vi "Create Logger.vi"(8 "error in (no error)":errorcluster, 11 "Logger.Error in":refnum<class "Logger.Error.lvclass">) -> (0 "error out":errorcluster, 3 "Logger.Error out":refnum<class "Logger.Error.lvclass">)   [LabVIEW 2016, in "Logger.Error.lvclass"]
uses:
  Logger.Error.lvclass
  <userlib>/_MGI/Error Reporter/MGI Error Reporter Base/MGI Error Reporter Base.lvclass
  <userlib>/_MGI/Error Reporter/MGI Error Reporter Dialog/MGI Error Reporter Dialog.lvclass
  Logger/Logger.lvclass
  C:/Program Files (x86)/National Instruments/LabVIEW 2016/user.lib/_MGI/Error Reporter/MGI Error Reporter Base/MGI Error Reporter Base.lvclass
panel:
  out "Already Running?":bool
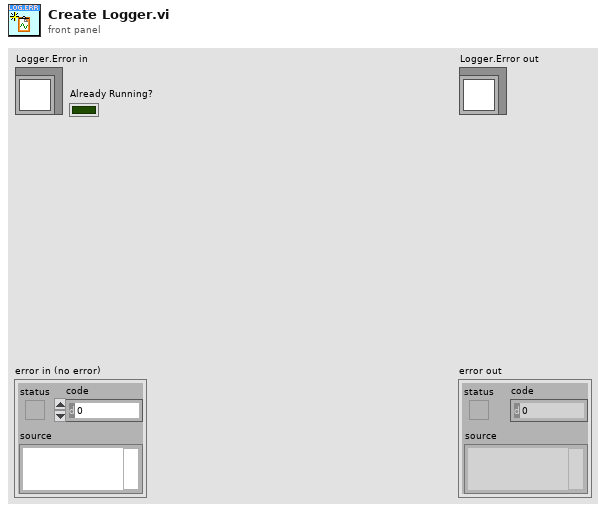
[diagram p1: front panel]
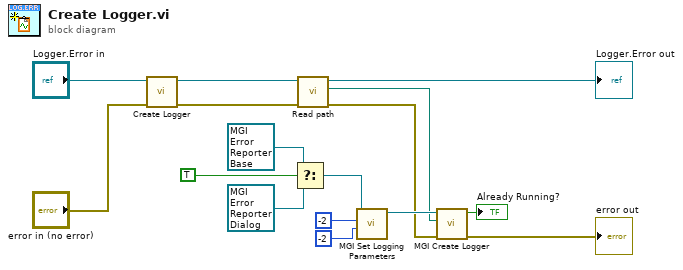
[diagram p0: block diagram]
diagram:
  n1 = call-parent "Create Logger.vi"("error in (no error)"="error in (no error)", "Logger in"="Logger.Error in") -> ("error out"=w5:errorcluster, "Logger out"=w4:refnum<class "Logger.Error.lvclass">)  [unwired: 8 in]
  n2 = Select(t=refnum<class "MGI Error Reporter Base.lvclass"> refnum ("MGI Error Reporter Base In"), s=TRUE, f=refnum<class "MGI Error Reporter Dialog.lvclass"> refnum ("Reporter Dialog.lvclass")) -> (s? t:f=w9:refnum<class "MGI Error Reporter Base.lvclass">)
  n3 = call-dynamic "Read path.vi"("error in (no error)"=w5, "Logger in"=w4) -> ("error out"=w6:errorcluster, "path"=w2:path, "Logger out"=→"Logger.Error out":refnum<class "Logger.Error.lvclass">)  [unwired: 7 in]
  n4 = call <userlib>:"MGI Set Logging Parameters.vi"("Max # Log Files (Don't change)"=-2, "Max # Errors to Log (Don't change)"=-2, "MGI Error Reporter Base In"=w9) -> ("MGI Error Reporter Base Out"=w14:refnum<class "MGI Error Reporter Base.lvclass">)  [unwired: 8 in]
  n5 = call <userlib>:"MGI Create Logger.vi"("error in (no error)"=w6, "Error Log Directory \n(Not a Path: Shared Docs\\Caller Prefix)\n(\"\" Path: Turn off logging)"=w2, "Error Reporter"=w14) -> ("error out"=→"error out":errorcluster, "Already Running?"=→"Already Running?":bool)  [unwired: 6 in, 1 out]
